vi "HostTestSimpleCounter.vi"() -> ()   [LabVIEW 2014]
uses:
  <vilib>/FPGAPlugInAG/PXI-7852R/niLvFpga_Open_PXI-7852R.vi
  <vilib>/rvi/interface/common/dynamic/niFpgaDynamicAddResources.vi
  <vilib>/Utility/error.llb/Error Cluster From Error Code.vi
  <vilib>/FPGAPlugInAG/Dynamic/niLvFpga_Run_Dynamic.vi
  <vilib>/rvi/errors/niLvFpgaAdjustHostInterfaceError.vi
  <vilib>/FPGAPlugInAG/Dynamic/niLvFpga_Close_Dynamic.vi
  <vilib>/rvi/interface/nirviOpenFPGA/nirviOpenFPGA.xnode
  FPGA Bitfiles/TiTaProj_DAF_SPMain_w3ru5+-JEpc.lvbitx
  <vilib>/rvi/interface/nirviMethod/nirviMethod.xnode
  <vilib>/rvi/interface/nirviReadWriteControl/nirviReadWriteControl.xnode
  <vilib>/rvi/interface/nirviCloseFPGA/nirviCloseFPGA.xnode
  <vilib>/FPGAPlugInAG/Dynamic/niLvFpga_ReadFifo_Dynamic.vi
  <vilib>/rvi/errors/niLvFpgaMergeErrorWithErrorCode.vi
  <vilib>/rvi/interface/Simulation/niFpgaSimulationCallBeginRW.vi
  <vilib>/FPGAPlugInAG/Dynamic/niLvFpga_StartFifo_Dynamic.vi
  NiFpgaLv.dll
panel:
  out "Overflow":bool
  out "floor(x/y)":u32
  out "output array":u32[](array[numeric]) format="%032b"
  out "Elements Remaining":u32
  in  "stop":bool
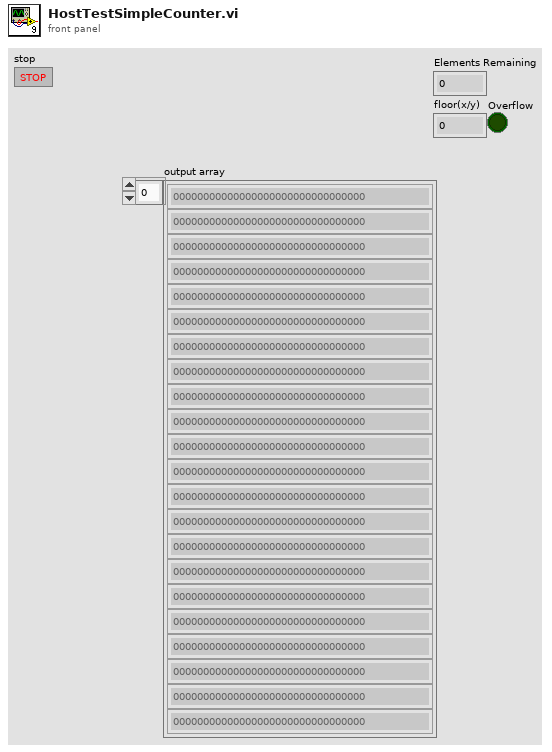
[diagram p1: front panel]
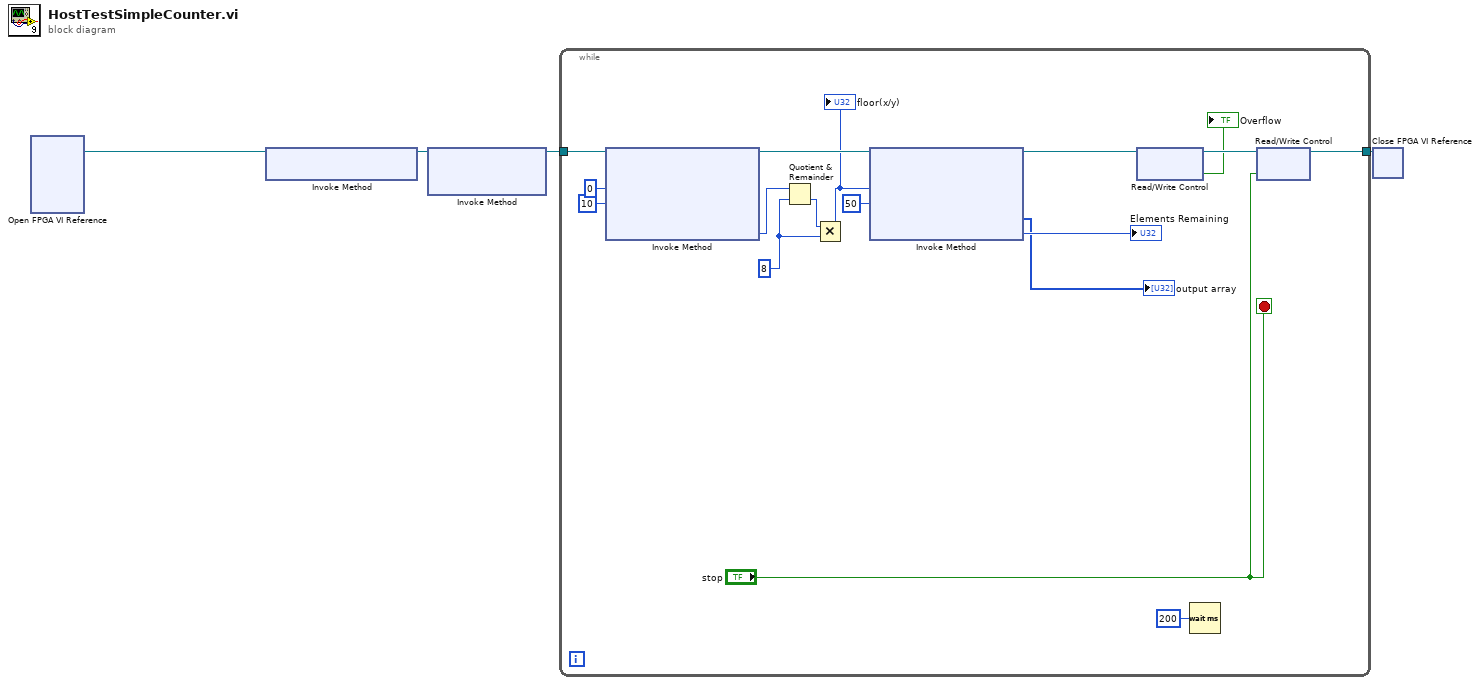
[diagram p0: block diagram]
diagram:
  n1 = xnode "Open FPGA VI Reference"() -> ("FPGA VI Reference Out"=w1:refnum<k20>)  [unwired: 2 in, 1 out]
  n2 = xnode "Invoke Method"("FPGA VI Reference In"=w1) -> ("FPGA VI Reference Out"=w3:refnum<k20>)  [unwired: 1 in, 1 out]
  n3 = xnode "Invoke Method"("FPGA VI Reference In"=w3) -> ("FPGA VI Reference Out"=w2:refnum<k20>)  [unwired: 2 in, 1 out]
  n4 = while {
    tunnel: w2 -> [w17]
    tunnel: [w18] -> w4
    stop <- "stop" stop-if-true
    w10 = u32 8 ("y")
    n5 = xnode "Invoke Method"("FPGA VI Reference In"=w17, "Number of Elements"=u32 0, "Timeout (ms)"=10) -> ("FPGA VI Reference Out"=w20:refnum<k20>, "Elements Remaining"=w15:u32)  [unwired: 1 in, 2 out]
    n6 = Quotient & Remainder(x=w15, y=w10) -> (floor(x/y)=w9:u32)  [unwired: 1 out]
    n7 = Multiply(x=w9, y=w10) -> (x*y=w5:u32)
    "floor(x/y)" <- w5
    n8 = xnode "Invoke Method"("FPGA VI Reference In"=w20, "Number of Elements"=w5, "Timeout (ms)"=50) -> ("FPGA VI Reference Out"=w19:refnum<k20>, "Data"=→"output array":u32[], "Elements Remaining"=→"Elements Remaining":u32)  [unwired: 1 in, 1 out]
    n9 = xnode "Read/Write Control"("FPGA VI Reference In"=w19) -> ("FPGA VI Reference Out"=w8:refnum<k20>, "Overflow"=→"Overflow":bool)  [unwired: 1 in, 1 out]
    n10 = Wait (ms)(milliseconds to wait=u32 200) -> ()  [unwired: 1 out]
    n11 = xnode "Read/Write Control"("FPGA VI Reference In"=w8, "stop"="stop") -> ("FPGA VI Reference Out"=w18:refnum<k20>)  [unwired: 1 in, 1 out]
  }
  n12 = xnode "Close FPGA VI Reference"("FPGA VI Reference In"=w4) -> ()  [unwired: 1 in, 1 out]
